vi "ImageEqualizer.vi"(8 "error in (no error)":errorcluster, 10 "axis to equalize":enum16{"X axis", "Y axis"}(ring), 11 "Image in":T1) -> (0 "error out":errorcluster, 3 "Image out":T1)   [LabVIEW 2012]
uses:
  <vilib>/vision/Image Controls.llb/IMAQ Image.ctl
  <vilib>/vision/NI_Vision_Development_Module.lvlib
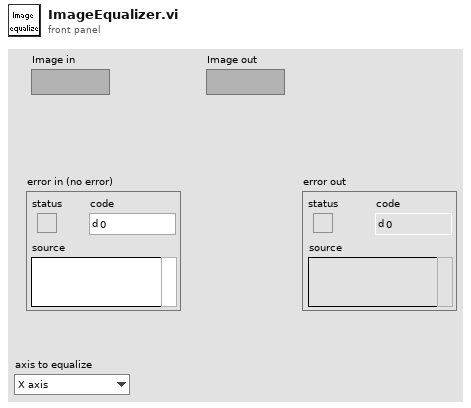
[diagram p1: front panel]
types:
  T1 = typedef "IMAQ Image.ctl" = refnum<image>
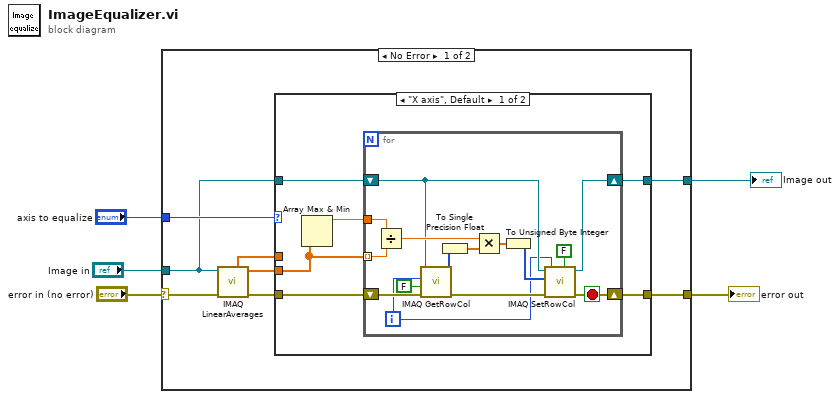
[diagram p0: block diagram]
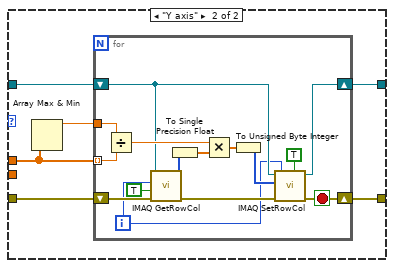
[diagram p2: hidden frame]
diagram:
  n1 = case shown="No Error" "error in (no error)" {
    selector: "error in (no error)" -> [w13 w56]
    tunnel: "Image in" -> [w8 w57]
    tunnel: "axis to equalize" -> [w12 _]
    tunnel: [w7 w57] -> w2
    tunnel: [w6 w56] -> w1
    frame No Error {
      n2 = call "IMAQ LinearAverages"("error in (no error)"=w13, "Image Src"=w8) -> ("error out"=w9:errorcluster, "Y Axis Averages"=w11:sgl[], "X Axis Averages"=w10:sgl[])  [unwired: 5 in, 2 out]
      n3 = case shown="\"X axis\", Default" w12 {
        tunnel: w11 -> [w14 _]
        tunnel: w10 -> [_ w40]
        tunnel: w9 -> [w17 w38]
        tunnel: w8 -> [w18 w37]
        tunnel: [w15 w36] -> w7
        tunnel: [w16 w35] -> w6
        frame "X axis", Default {
          n4 = Array Max & Min(array=w14) -> (max value=w19:sgl)  [unwired: 3 out]
          n5 = for {
            tunnel: w14 -> [w33] mode=indexing
            tunnel: w19 -> [w34]
            shift-right: [w20] -> w16
            shift-left: w17 -> [w32]
            shift-right: [w23] -> w15
            shift-left: w18 -> [w24]
            i -> [w22]
            stop <- w20 stop-if-true
            n6 = Divide(x=w34, y=w33) -> (x/y=w28:sgl)
            n7 = call "IMAQ GetRowCol"("Image"=w24, "Number"=w22, "Row / Column (Row)"=FALSE, "error in (no error)"=w32) -> ("Pixels (U8)"=w30:u8[], "error out"=w25:errorcluster)  [unwired: 2 in, 3 out]
            n8 = To Single Precision Float(number=w30) -> (single precision float=w29:sgl[])
            n9 = Multiply(x=w28, y=w29) -> (x*y=w27:sgl[])
            n10 = To Unsigned Byte Integer(number=w27) -> (unsigned 8bit integer=w26:u8[])
            n11 = call "IMAQ SetRowCol"("Row / Column (Row)"=FALSE, "Number"=w22, "error in (no error)"=w25, "Pixels (U8)"=w26, "Image"=w24) -> ("error out"=w20:errorcluster, "Image Out"=w23:T1)  [unwired: 5 in]
          }
        }
        frame "Y axis" {
          n12 = Array Max & Min(array=w40) -> (max value=w39:sgl)  [unwired: 3 out]
          n13 = for {
            tunnel: w40 -> [w54] mode=indexing
            tunnel: w39 -> [w55]
            shift-right: [w41] -> w35
            shift-left: w38 -> [w53]
            shift-right: [w44] -> w36
            shift-left: w37 -> [w45]
            i -> [w43]
            stop <- w41 stop-if-true
            n14 = Divide(x=w55, y=w54) -> (x/y=w49:sgl)
            n15 = call "IMAQ GetRowCol"("Image"=w45, "Number"=w43, "Row / Column (Row)"=TRUE, "error in (no error)"=w53) -> ("Pixels (U8)"=w51:u8[], "error out"=w46:errorcluster)  [unwired: 2 in, 3 out]
            n16 = To Single Precision Float(number=w51) -> (single precision float=w50:sgl[])
            n17 = Multiply(x=w49, y=w50) -> (x*y=w48:sgl[])
            n18 = To Unsigned Byte Integer(number=w48) -> (unsigned 8bit integer=w47:u8[])
            n19 = call "IMAQ SetRowCol"("Row / Column (Row)"=TRUE, "Number"=w43, "error in (no error)"=w46, "Pixels (U8)"=w47, "Image"=w45) -> ("error out"=w41:errorcluster, "Image Out"=w44:T1)  [unwired: 5 in]
          }
        }
      }
    }
    frame Error {
    }
  }
  "Image out" <- w2
  "error out" <- w1
